vi "read_system_clock.vi"() -> (0 "Total Seconds from Midnight":dbl format="%.4f", 1 "output string":string="Frame time stamp: \tJanuary 23 2007: 12:12:34:.9818\r\n", 2 "LABVIEW TIME STAMP":timestamp=timestamp(3258559454.312 s since 1904-01-01) format="%<%.4X\n%x>T")   [LabVIEW 2014]
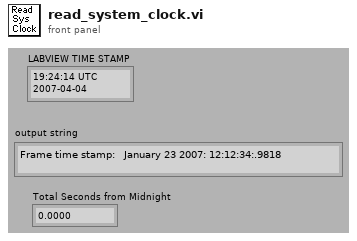
[diagram p1: front panel]
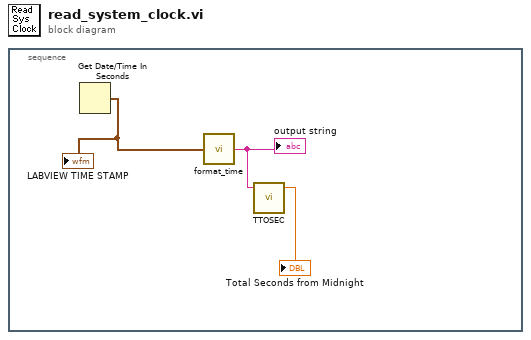
[diagram p0: block diagram]
diagram:
  n1 = stacked-sequence {
    frame #0 {
      n2 = Get Date/Time In Seconds() -> (seconds since 1Jan1904=w3:timestamp)
      "LABVIEW TIME STAMP" <- w3
      n3 = call "format_time.vi"("Frame Time Stamp"=w3) -> ("output string"=w2:string)
      "output string" <- w2
      n4 = call "TTOSEC.VI"("String"=w2) -> ("Total Seconds from Midnight"=→"Total Seconds from Midnight":dbl)  [unwired: 1 in, 3 out]
    }
  }
